vi "Main.vi"() -> ()   [LabVIEW 2018]
uses:
  <vilib>/myRIO/Instrument Drivers/Onboard IO/DIO/vis/Write.vi
  <vilib>/myRIO/Instrument Drivers/Onboard IO/SPI/vis/Configure.vi
  <vilib>/myRIO/Instrument Drivers/Onboard IO/SPI/vis/Read.vi
  <vilib>/myRIO/Common/Instrument Driver Framework/myRIO v1.0/UART/vis/myRIO v1.0 Close UART.vi
  <vilib>/myRIO/Instrument Drivers/Onboard IO/SPI/vis/Write Read.vi
  <vilib>/myRIO/Instrument Drivers/Onboard IO/DIO/vis/Smart Open.vi
  <vilib>/Utility/error.llb/Error Cluster From Error Code.vi
  <vilib>/myRIO/Common/Instrument Driver Framework/myRIO v1.0/DIO/vis/myRIO v1.0 Write DIO.vi
  <vilib>/myRIO/Instrument Drivers/Onboard IO/SPI/vis/Smart Open.vi
  <vilib>/myRIO/Common/Instrument Driver Framework/myRIO v1.0/SPI/vis/myRIO v1.0 Configure SPI.vi
  <vilib>/myRIO/Common/Instrument Driver Framework/myRIO v1.0/SPI/vis/myRIO v1.0 Write Read SPI.vi
  <vilib>/myRIO/Common/Instrument Driver Framework/Utilities/vis/FPGA Ref Manager.vi
  <vilib>/myRIO/Common/Instrument Driver Framework/myRIO v1.0/myRIO v1.0 Reset FPGA.vi
  <vilib>/myRIO/Common/Instrument Driver Framework/myRIO v1.0/IRQ/vis/myRIO v1.0 IRQ Info FGV.vi
  <vilib>/myRIO/Common/Instrument Driver Framework/myRIO v1.0/IRQ/vis/myRIO v1.0 Timer IRQ Info FGV.vi
  <vilib>/myRIO/Common/Instrument Driver Framework/myRIO v1.0/IRQ/vis/myRIO v1.0 ISR Agent.vi
  <vilib>/myRIO/Instrument Drivers/Utilities/Utilities.lvlib
panel:
  out "x/y":dbl
  out "sensor value":u8(knob) scale=0.0..255.0
  in  "[ESC]":bool
  # "Ambient Light Sensor demo"
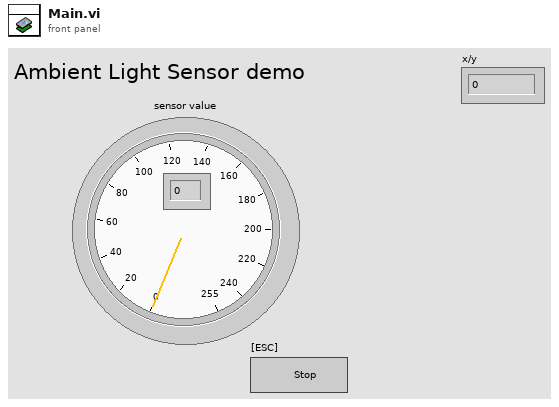
[diagram p1: front panel]
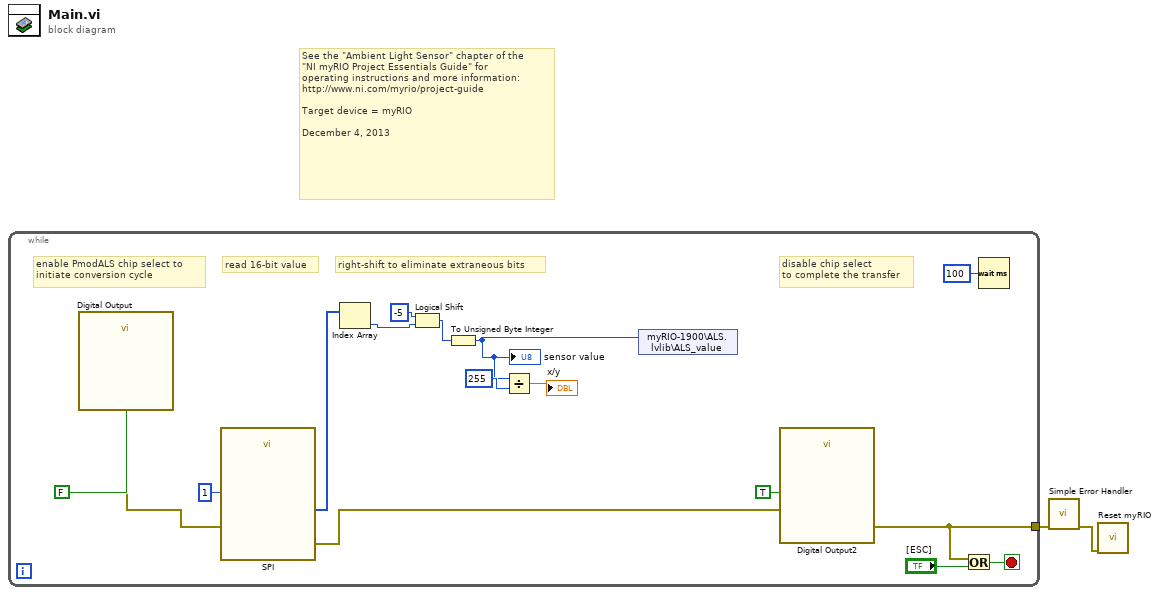
[diagram p0: block diagram]
diagram:
  # "See the \"Ambient Light Sensor\" chapter of the\n\"NI myRIO Project Essentials Guide\" for\noperating instructions and more information: \nhttp://www.ni.com/myrio/project-guide\n\nTarget device = myRIO\n\nDecember 4, 2013"
  n1 = while {
    tunnel: [w11] -> w2
    stop <- w18 stop-if-true
    # "right-shift to eliminate extraneous bits"
    # "disable chip select\nto complete the transfer"
    # "read 16-bit value"
    # "enable PmodALS chip select to\ninitiate conversion cycle"
    n2 = call "Digital Output"("B/DIO0 (Pin 11)"=FALSE ("A/DIO0 (Pin 11)")) -> ("error out"=w14:errorcluster)  [unwired: 26 in]
    n3 = call "SPI"("Frame Count"=u32 1, "error in (no error)"=w14) -> ("Frames Read"=w9:u16[], "error out"=w12:errorcluster)  [unwired: 24 in]
    n4 = Index Array "Index Array"(array=w9) -> (element=w8:u16)  [unwired: 1 in]
    n5 = Logical Shift(y=i16 -5, x=w8) -> (x << y=w6:u16)
    n6 = To Unsigned Byte Integer(number=w6) -> (unsigned 8bit integer=w3:u8)
    "sensor value" <- w3
    n7 = Divide(x=w3, y=u8 255 ("x")) -> (x/y=→"x/y":dbl)
    n8 = shared-variable "myRIO-1900\\ALS.lvlib\\ALS_value"(w3) -> ()  [unwired: 1 in, 1 out]
    n9 = call "Digital Output2"("B/DIO0 (Pin 11)"=TRUE ("A/DIO0 (Pin 11)"), "error in (no error)"=w12) -> ("error out"=w11:errorcluster)  [unwired: 25 in]
    n10 = Or(x=w11, y="[ESC]") -> (x .or. y?=w18:bool)
    n11 = Wait (ms)(milliseconds to wait=u32 100) -> ()  [unwired: 1 out]
  }
  n12 = call <vilib>:"Simple Error Handler.vi"("error in (no error)"=w2) -> ("error out"=w1:errorcluster)  [unwired: 4 in, 4 out]
  n13 = call <vilib>:"Reset myRIO.vi"("error in (no error)"=w1) -> ()  [unwired: 10 in, 1 out]
